vi "Determine Warnings.vi"(8 "Error In":errorcluster) -> (0 "Error Out":errorcluster)   [LabVIEW 2019]
panel:
  out "Warning Text":string
  out "Warning?":bool
  in  "Min Temperature":dbl
  in  "Max Temperature":dbl
  in  "Current Temperature":dbl
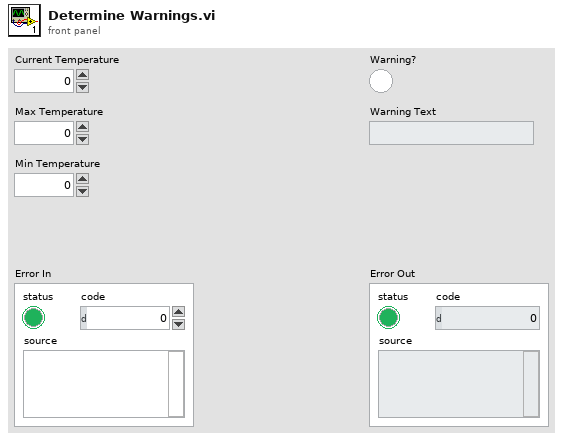
[diagram p1: front panel]
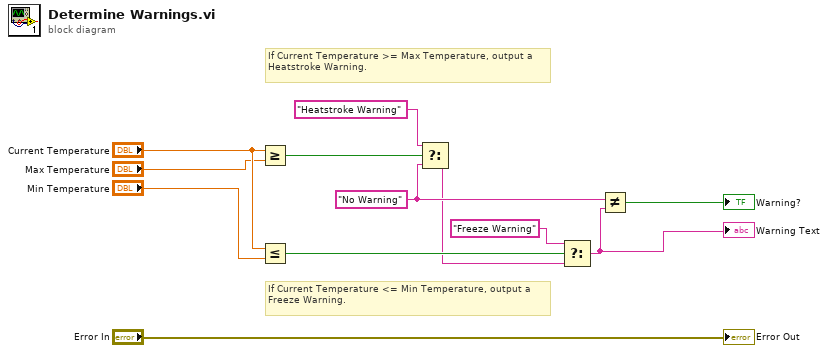
[diagram p0: block diagram]
diagram:
  w9 = "No Warning"
  # "If Current Temperature <= Min Temperature, output a Freeze Warning."
  # "If Current Temperature >= Max Temperature, output a Heatstroke Warning."
  n1 = Greater Or Equal?(x="Current Temperature", y="Max Temperature") -> (x >= y?=w12:bool)
  n2 = Less Or Equal?(x="Current Temperature", y="Min Temperature") -> (x <= y?=w10:bool)
  n3 = Select(t="Heatstroke Warning", s=w12, f=w9) -> (s? t:f=w8:string)
  n4 = Select(t="Freeze Warning", s=w10, f=w8) -> (s? t:f=w1:string)
  "Warning Text" <- w1
  n5 = Not Equal?(x=w9, y=w1) -> (x != y?=→"Warning?":bool)
  "Error Out" <- "Error In"
